vi "heatmap_lines_producer.vi"() -> ()   [LabVIEW 2015]
uses:
  <vilib>/Utility/file.llb/Read Delimited Spreadsheet (DBL).vi
panel:
  out "Intensity Graph 2":dbl[][](graph)
  in  "Path":path=path "C:/Users/arnold/Documents/labview/afm_imaging/grating01.csv"
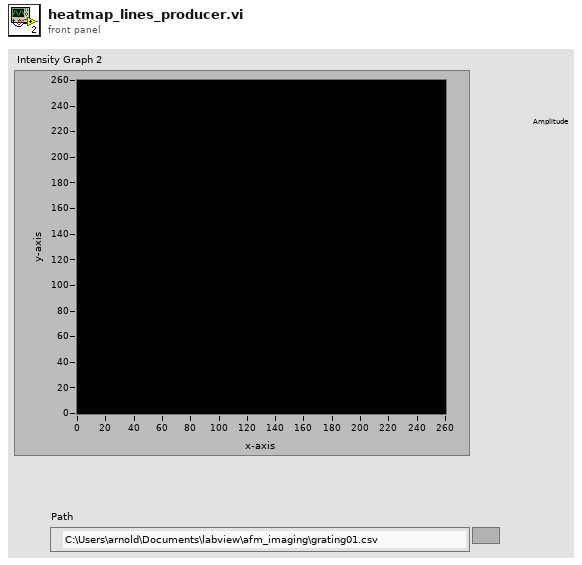
[diagram p1: front panel]
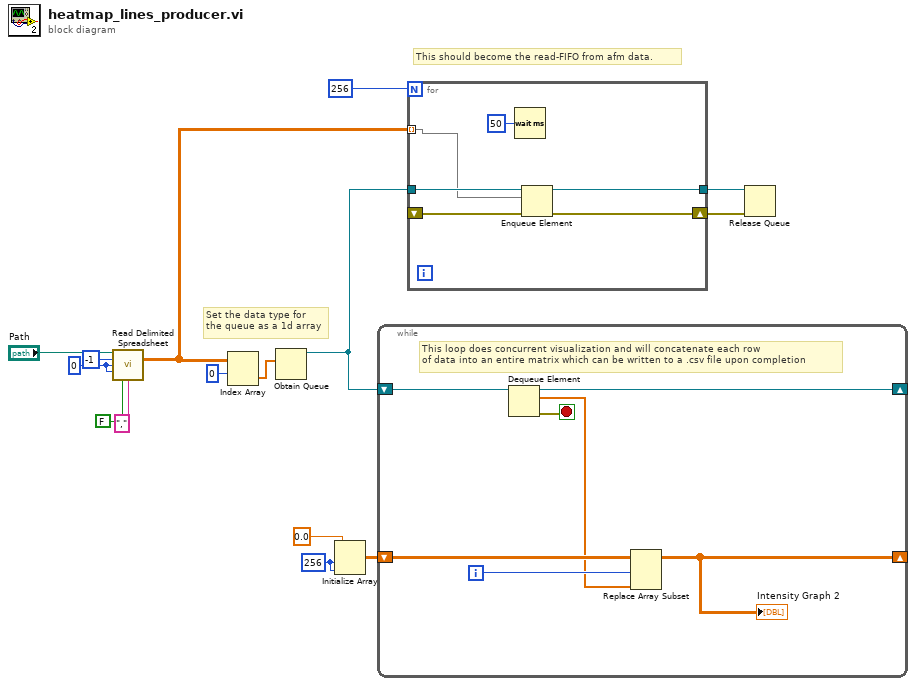
[diagram p0: block diagram]
diagram:
  w10 = 256 ("dimension size")
  w12 = 0 ("start of read offset (chars.:0)")
  # "Set the data type for\nthe queue as a 1d array"
  # "This should become the read-FIFO from afm data."
  n1 = call-poly <vilib>:"Read Delimited Spreadsheet.vi"("file path (dialog if empty)"="Path", "number of rows (all:-1)"=-1, "start of read offset (chars.:0)"=w12, "max characters/row  (no limit:0)"=w12, "transpose? (F)"=FALSE, "delimiter (\\t)"="," ("delimiter (\\t)")) -> ("all rows"=w1:dbl[][])  [unwired: 4 in, 5 out]
  n2 = Index Array(array=w1, index (row)=0) -> (element=w2:dbl[])  [unwired: 1 in]
  n3 = Obtain Queue(element data type=w2) -> (queue out=w6:refnum<queue>)  [unwired: 4 in, 2 out]
  n4 = Initialize Array(0.0 ("element"), w10, w10) -> (w8:dbl[][])
  n5 = while {
    shift-right: [w21] -> _
    shift-left: w6 -> [w22]
    shift-right: [w18] -> _
    shift-left: w8 -> [w19]
    i -> [w20]
    stop <- w16 stop-if-true
    # "This loop does concurrent visualization and will concatenate each row \nof data into an entire matrix which can be written to a .csv file upon completion"
    n6 = Dequeue Element(queue=w22) -> (queue out=w21:refnum<queue>, element=w17:dbl[], error out=w16:errorcluster)  [unwired: 2 in, 1 out]
    n7 = Replace Array Subset(array=w19, new element=w17, index (row)=w20) -> (w18:dbl[][])  [unwired: 1 in]
    "Intensity Graph 2" <- w18
  }
  n8 = for {
    N: 256 -> [_]
    tunnel: w1 -> [w23] mode=indexing
    tunnel: w6 -> [w28]
    tunnel: [w27] -> w5
    shift-right: [w26] -> w4
    shift-left: _ -> [w25]
    n9 = Wait (ms)(milliseconds to wait=u32 50) -> ()  [unwired: 1 out]
    n10 = Enqueue Element(queue=w28, element=w23, error in (no error)=w25) -> (queue out=w27:refnum<queue>, error out=w26:errorcluster)  [unwired: 1 in, 1 out]
  }
  n11 = Release Queue(queue=w5, error in (no error)=w4) -> ()  [unwired: 1 in, 3 out]
